vi "Altimeter.vi"() -> (3 "Altitude":dbl)   [LabVIEW 2015]
uses:
  BMP085 (GY-65) Library/BMP085 (RT).lvlib
panel:
  out "Uncertainty Range":dbl
  out "Min Recorded":dbl
  out "Max Recorded":dbl
  out "History 2":cluster{"Temp [°C]":dbl, "hPa":dbl}(graph)
  out "Temperature [°C] 2":dbl(slide) scale=0.0..80.0
  out "Pressure [hPa]":dbl(knob) scale=900.0..1100.0
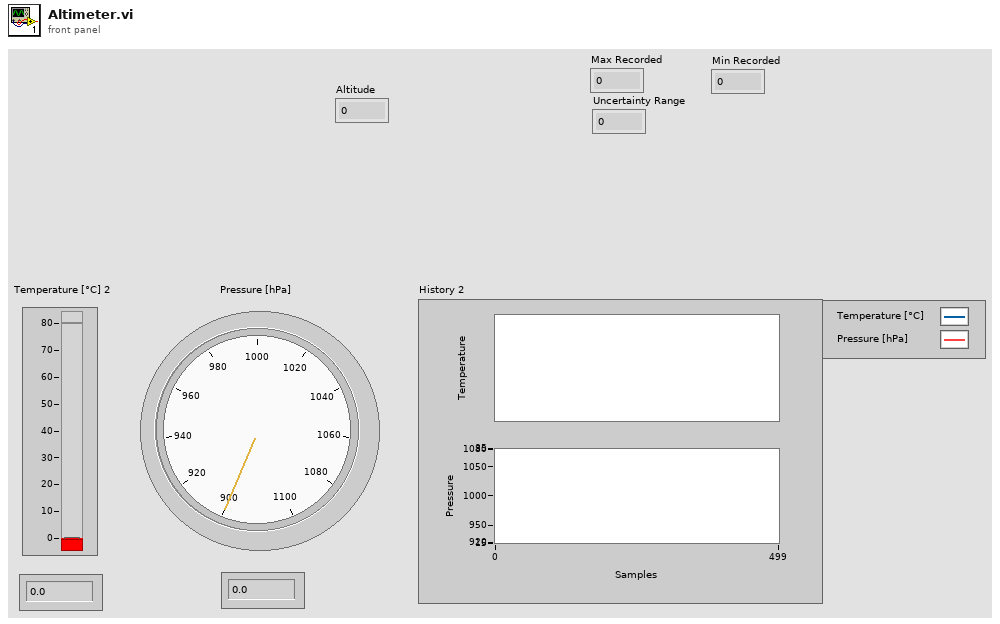
[diagram p1: front panel]
types:
  T1 = enum8{"ultra low power", "standard", "high resolution", "ultra high resolution"}
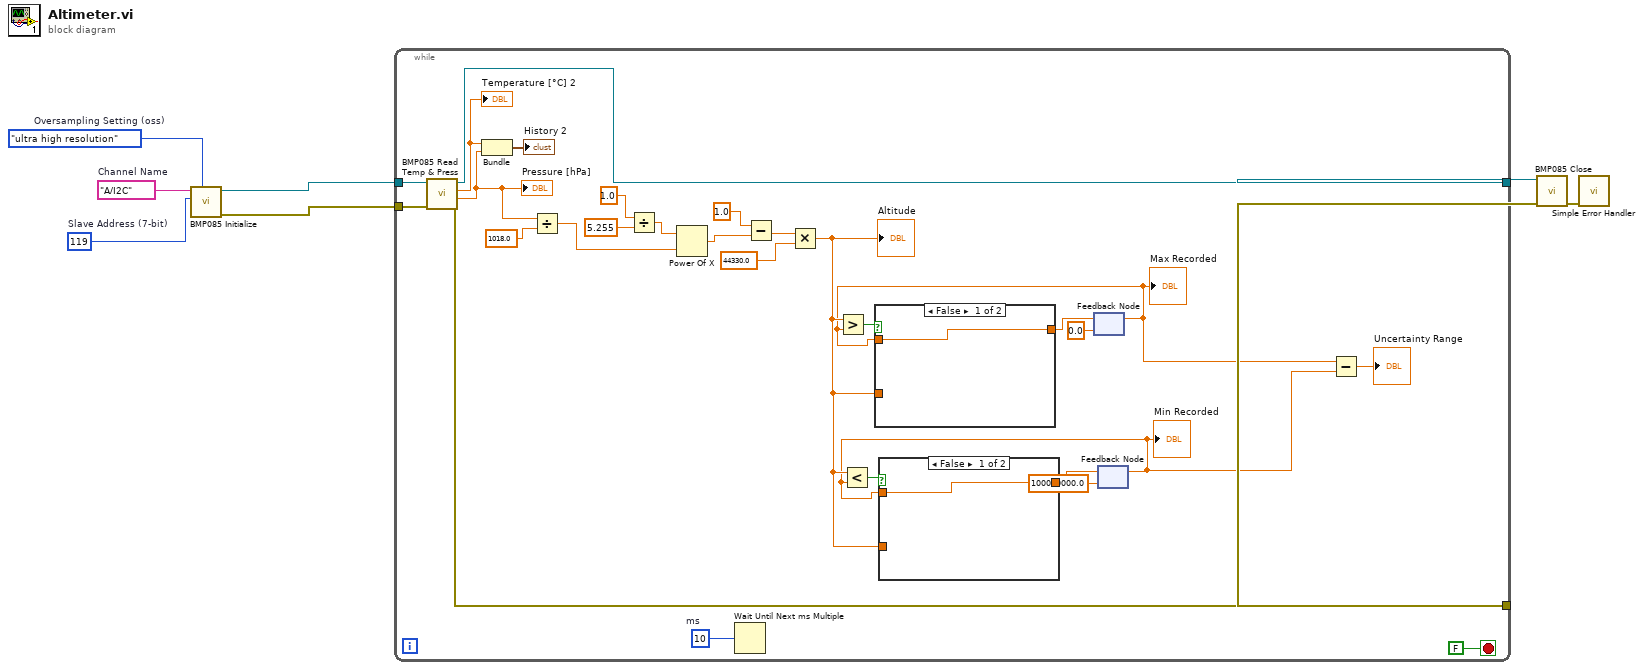
[diagram p0: block diagram]
diagram:
  w6 = u8 119  # Slave Address (7-bit)
  w7 = T1."ultra high resolution"  # Oversampling Setting (oss)
  w8 = tag "A/I2C"  # Channel Name
  n1 = call "BMP085 Initialize.vi"("Oversampling Setting (oss)"=w7, "Slave Address (7-bit)"=w6, "Channel Name"=w8) -> ("error out"=w5:errorcluster, "BMP085 (GY-65) out"=w4:refnum<class "BMP085 (GY-65).lvclass">)  [unwired: 7 in]
  n2 = while {
    tunnel: w5 -> [w33]
    tunnel: w4 -> [w32]
    tunnel: [w31] -> w2
    tunnel: [w30] -> w1
    stop <- FALSE stop-if-true
    w36 = u32 10  # ms
    n3 = call "BMP085 Read Temp & Press.vi"("error in (no error)"=w33, "BMP085 (GY-65) in"=w32) -> ("error out"=w31:errorcluster, "hPa"=w28:dbl, "Temp [°C]"=w35:dbl, "BMP085 (GY-65) out"=w30:refnum<class "BMP085 (GY-65).lvclass">)  [unwired: 6 in]
    "Pressure [hPa]" <- w28
    "Temperature [°C] 2" <- w35
    n4 = Bundle("Temp [°C]"=w35, "hPa"=w28) -> (→"History 2":cluster{"Temp [°C]":dbl, "hPa":dbl})  [unwired: 1 in]
    n5 = Divide(x=w28, y=1018.0) -> (x/y=w26:dbl)
    n6 = Divide(x=1.0, y=5.255) -> (x/y=w25:dbl)
    n7 = Power Of X(1:w26, 2:w25) -> (0:w22:dbl)
    n8 = Wait Until Next ms Multiple(millisecond multiple=w36) -> ()  [unwired: 1 out]
    n9 = Subtract(x=1.0, y=w22) -> (x-y=w20:dbl)
    n10 = Multiply(x=w20, y=44330.0) -> (x*y=w12:dbl)
    "Altitude" <- w12
    n11 = feedback #1(0.0) -> (w11:dbl)
    "Max Recorded" <- w11
    n12 = Greater?(x=w12, y=w11) -> (0:w18:bool)
    n13 = case shown="False" w18 {
      tunnel: w12 -> [_ w40]
      tunnel: [w39 w40] -> w17
      tunnel: w11 -> [w39 _]
      frame False {
      }
      frame True {
      }
    }
    n14 = feedback-in #1(w17) -> ()
    n15 = feedback #2(100000000.0) -> (w10:dbl)
    "Min Recorded" <- w10
    n16 = Less?(x=w12, y=w10) -> (x < y?=w15:bool)
    n17 = case shown="False" w15 {
      tunnel: w12 -> [_ w38]
      tunnel: [w37 w38] -> w14
      tunnel: w10 -> [w37 _]
      frame False {
      }
      frame True {
      }
    }
    n18 = feedback-in #2(w14) -> ()
    n19 = Subtract(x=w11, y=w10) -> (x-y=→"Uncertainty Range":dbl)
  }
  n20 = call "BMP085 Close.vi"("error in (no error)"=w2, "BMP085 (GY-65) in"=w1) -> ("error out"=w3:errorcluster)  [unwired: 9 in]
  n21 = call <vilib>:"Simple Error Handler.vi"("error in (no error)"=w3) -> ()  [unwired: 4 in, 5 out]
